vi "Open Waveform Sessions.vi"(8 "error in":errorcluster, 11 "Parameters":T4={"Name"="", "Rate.Hz"=0, "Injectors.Count"=0, "Injector.Timeout"=0.0, "Injector.Timer"=[], "Injector.Info"=[], "Events.Count"=[], "Event.Parameters"={"Shots"=0, "Shot.InitialVoltage"=0.0, "Shot.Stages"=0, "Stages"=[{"Stage.Dwell.Level"=0.0, "PullIn.Type"=enum."Pull In Transition Dwells", "PullIn.Level"=0.0, "Transition.Type"=enum."Stage Transition Voltage Level", "Transition.Level"=0.0}]}, "DMA.Ref"=refnum, "Waveform.Refs"=[], "Waveform.Sessions"=[], "Waveform.Enable"=refnum, "FPGA.Status"=refnum, "Search.Data"=refnum, "Results.Data"=refnum, "Results.Values"=[], "Results.Selections"=[]}) -> (0 "error out":errorcluster, 2 "Injection.Results":T1 {"Shots"."Results"."Off-Stage Avg Current" format="%#.6g"; "Shots"."Results"."Total Voltage Pulses" format="%#.6g"; "Shots"."Results"."Off-Stage Min Current" format="%#.6g"; "Shots"."Results"."Off-Stage Max Current" format="%#.6g"}, 3 "Parameters":T4={"Name"="", "Rate.Hz"=0, "Injectors.Count"=0, "Injector.Timeout"=0.0, "Injector.Timer"=[], "Injector.Info"=[], "Events.Count"=[], "Event.Parameters"={"Shots"=0, "Shot.InitialVoltage"=0.0, "Shot.Stages"=0, "Stages"=[{"Stage.Dwell.Level"=0.0, "PullIn.Type"=enum."Pull In Transition Dwells", "PullIn.Level"=0.0, "Transition.Type"=enum."Stage Transition Voltage Level", "Transition.Level"=0.0}]}, "DMA.Ref"=refnum, "Waveform.Refs"=[], "Waveform.Sessions"=[], "Waveform.Enable"=refnum, "FPGA.Status"=refnum, "Search.Data"=refnum, "Results.Data"=refnum, "Results.Values"=[], "Results.Selections"=[]})   [LabVIEW 2015, in "Fuel Injection Addon Engine.lvlib"]
uses:
  Fuel Injection Addon Engine.lvlib
  Types/Async Parameters.ctl
  Shared/Types/Injector info.ctl
  Shared/Types/Shot.Parameters.ctl
  Shared/Types/Stage.Parameters.ctl
  Shared/Types/Stage.PullIn.Types.ctl
  Shared/Types/Stage.Transition.Types.ctl
  <vilib>/NI Veristand/Custom Device API/Waveform Data Reference.ctl
  <vilib>/NI VeriStand/Custom Device Waveform API/Single Waveform Write (DBL)/Single Waveform Write (DBL).lvclass
  <vilib>/NI/NIVS Inline Async API/_Data Access Engine/Data Access Engine/Types/Read.DVR.ctl
  <vilib>/NI/NIVS Inline Async API/_Data Access Engine/Access Type Classes/Read/Read.lvclass
  <vilib>/NI/NIVS Inline Async API/_Data Access Engine/Data Access Engine/Types/Write.DVR.ctl
  <vilib>/NI/NIVS Inline Async API/_Data Access Engine/Access Type Classes/Write/Write.lvclass
  Shared/Types/Analysis.Channels.Select.ctl
  Types/Injector Event Data Cluster.ctl
  RT Analysis/Controls/Shot Information Control.ctl
  Types/Boost Stage Current Measurements Cluster Control.ctl
  <vilib>/NI Veristand/Custom Device Waveform API/Communication Properties.ctl
  <vilib>/NI Veristand/Custom Device Waveform API/Single Waveform Write (DBL)/NI VeriStand - Open Single Waveform Write Session (DBL).vi
  Shared/Constants.vi
  <vilib>/NI Veristand/Custom Device Waveform API/NI_VS Custom Device Waveform API.lvlib
  Shared/Fuel Injection Addon Shared.lvlib
  <vilib>/NI VeriStand/Custom Device API/Custom Device API.lvlib
  <vilib>/NI/NIVS Inline Async API/_Data Access Engine/Data Access Engine/Data Access Engine.lvclass
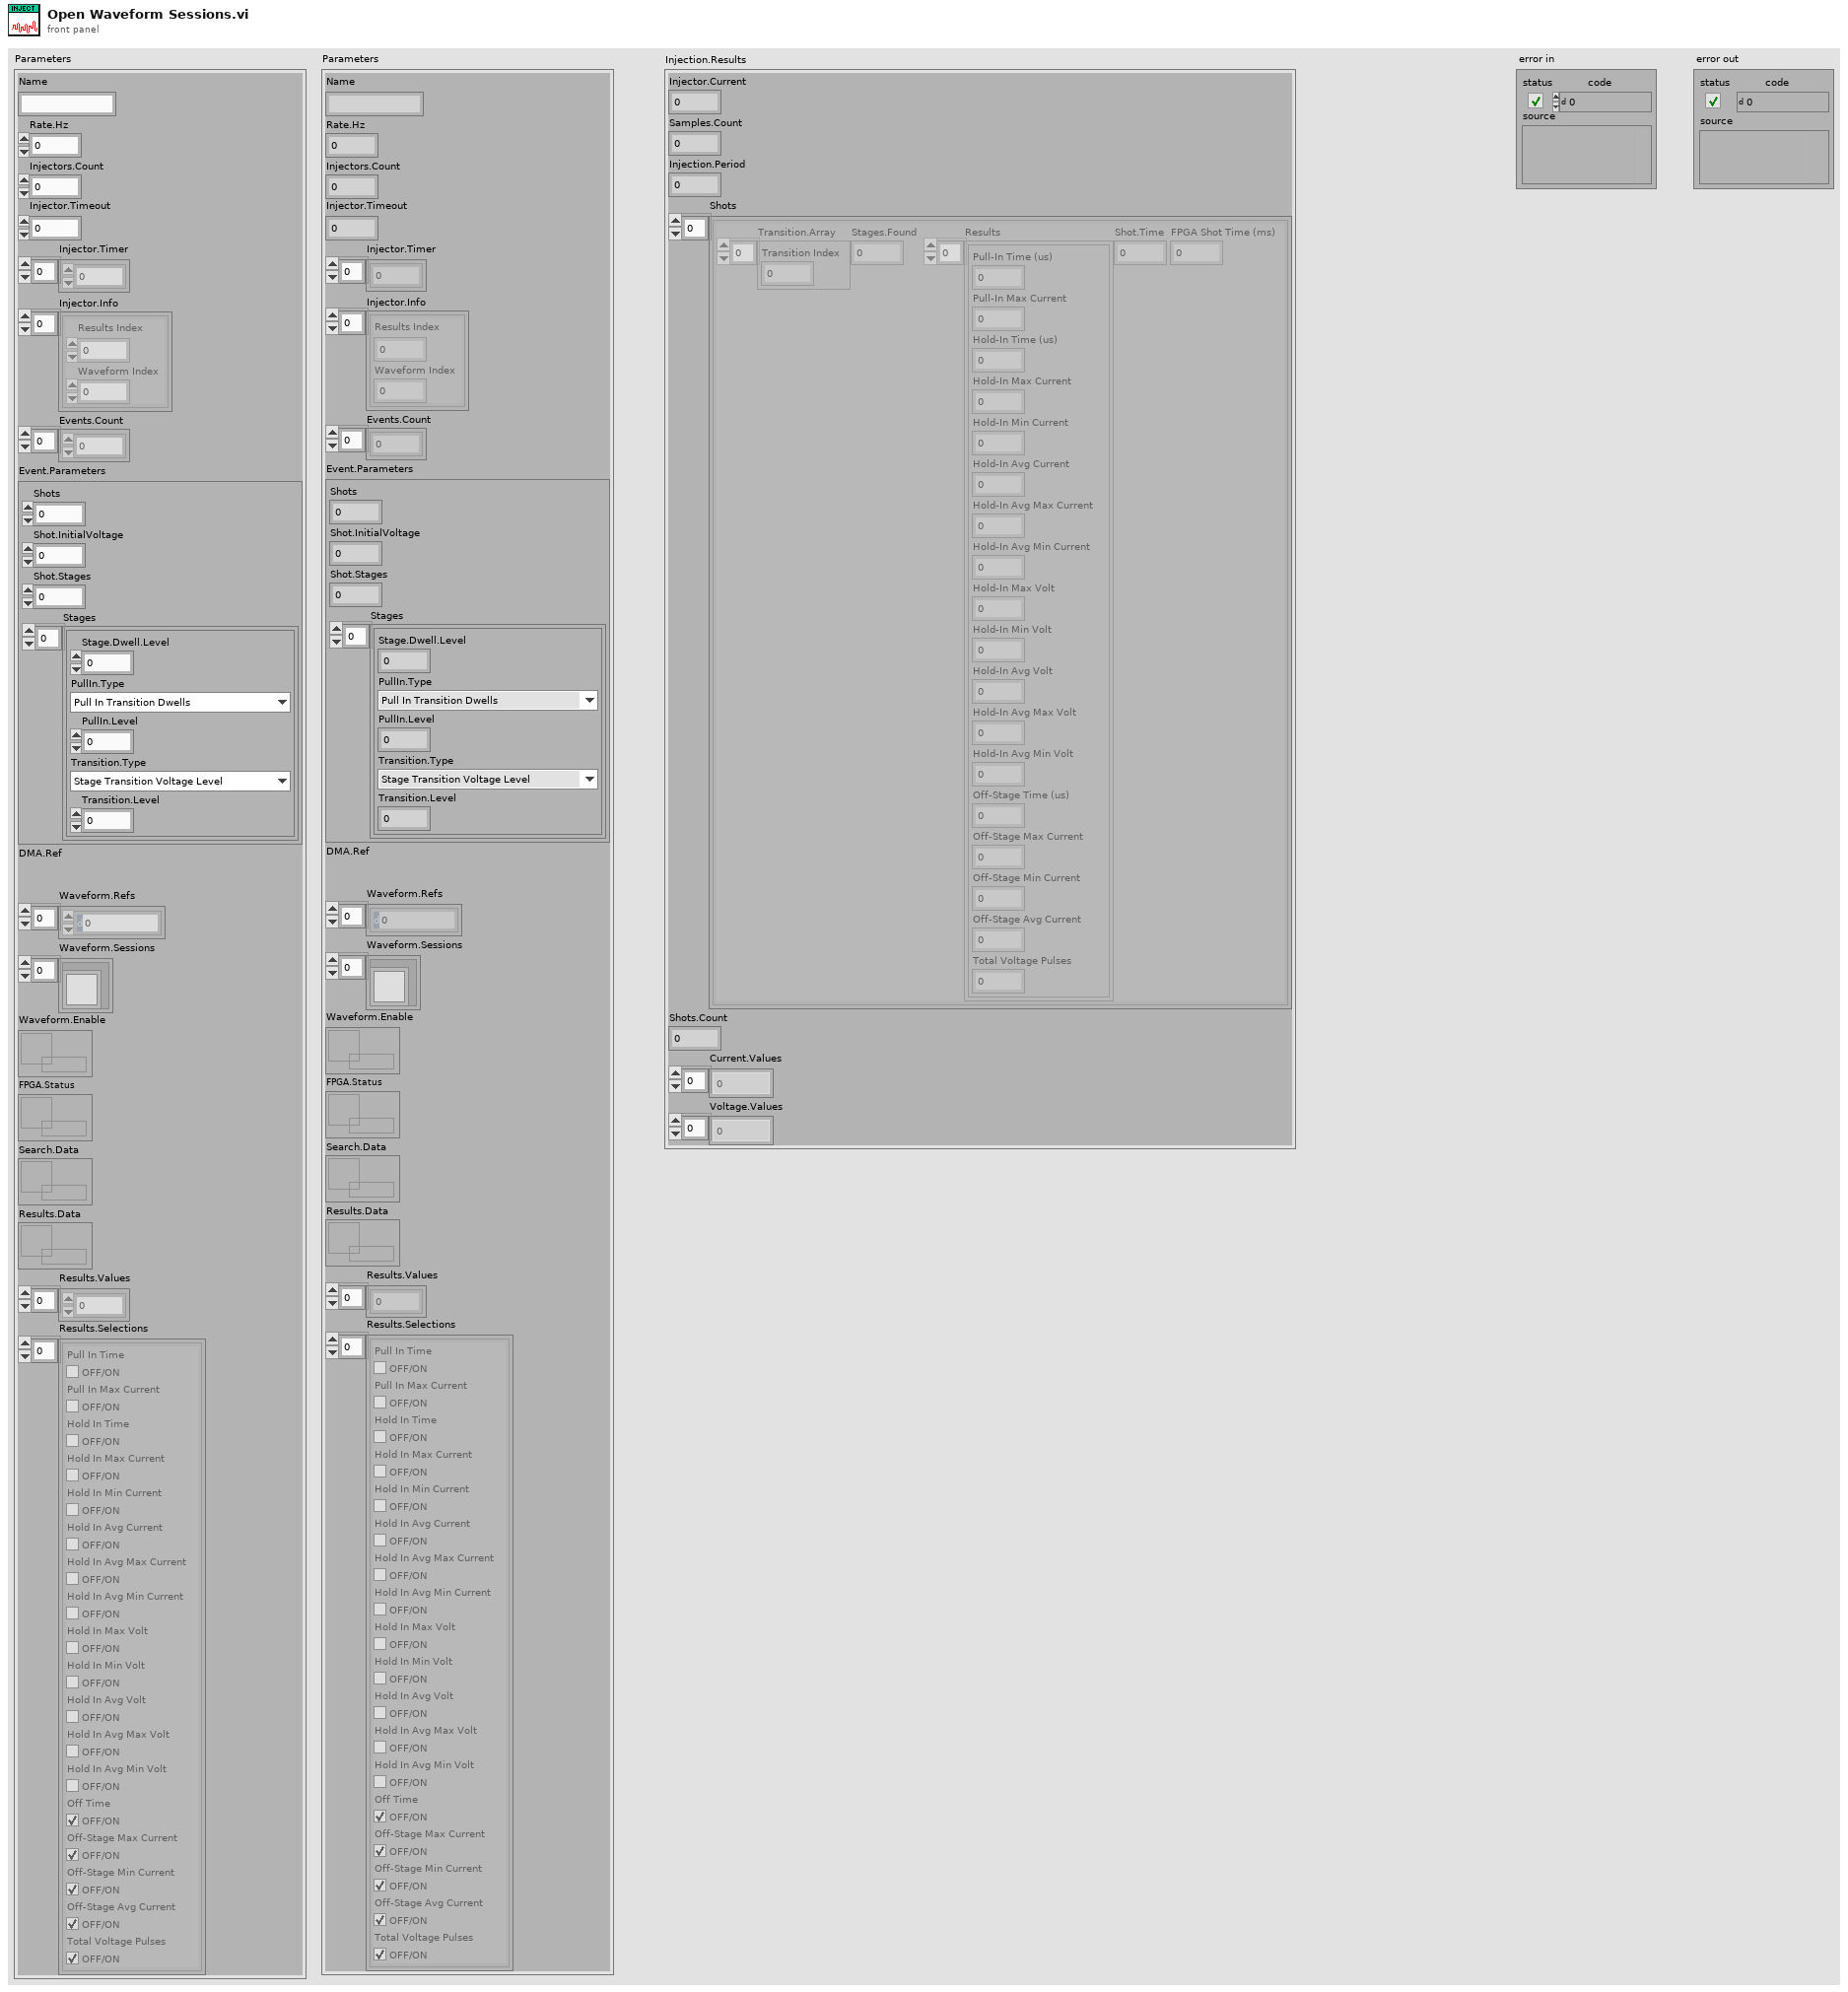
[diagram p1: front panel]
types:
  T1 = typedef "Fuel Injection Addon Engine.lvlib/Injector Event Data Cluster.ctl" = cluster{"Injector.Current":i16, "Samples.Count":i32, "Injection.Period":dbl, "Shots":T2[], "Shots.Count":i32, "Current.Values":dbl[], "Voltage.Values":dbl[]}
  T2 = typedef "Fuel Injection Addon Engine.lvlib/Shot Information Control.ctl" = cluster{"Transition.Array":i32[], "Stages.Found":u16, "Results":T3[], "Shot.Time":dbl, "FPGA Shot Time (ms)":dbl}
  T3 = typedef "Fuel Injection Addon Engine.lvlib/Boost Stage Current Measurements Cluster Control.ctl" = cluster{"Pull-In Time (us)":dbl, "Pull-In Max Current":dbl, "Hold-In Time (us)":dbl, "Hold-In Max Current":dbl, "Hold-In Min Current":dbl, "Hold-In Avg Current":dbl, "Hold-In Avg Max Current":dbl, "Hold-In Avg Min Current":dbl, "Hold-In Max Volt":dbl, "Hold-In Min Volt":dbl, "Hold-In Avg Volt":dbl, "Hold-In Avg Max Volt":dbl, "Hold-In Avg Min Volt":dbl, "Off-Stage Time (us)":dbl, "Off-Stage Max Current":dbl, "Off-Stage Min Current":dbl, "Off-Stage Avg Current":dbl, "Total Voltage Pulses":dbl}
  T4 = typedef "Fuel Injection Addon Engine.lvlib/Async Parameters.ctl" = cluster{"Name":string, "Rate.Hz":u32, "Injectors.Count":u8, "Injector.Timeout":dbl, "Injector.Timer":u32[], "Injector.Info":T5[], "Events.Count":u64[], "Event.Parameters":T6, "DMA.Ref":refnum<k20>, "Waveform.Refs":T10[], "Waveform.Sessions":refnum<class "Single Waveform Write (DBL).lvclass">[], "Waveform.Enable":T11, "FPGA.Status":T12, "Search.Data":T11, "Results.Data":T12, "Results.Values":dbl[], "Results.Selections":T13[]}
  T5 = typedef "Fuel Injection Addon Shared.lvlib/Injector info.ctl" = cluster{"Results Index":i32, "Waveform Index":i32}
  T6 = typedef "Fuel Injection Addon Shared.lvlib/Shot.Parameters.ctl" = cluster{"Shots":u32, "Shot.InitialVoltage":dbl, "Shot.Stages":u32, "Stages":T7[]}
  T7 = typedef "Fuel Injection Addon Shared.lvlib/Stage.Parameters.ctl" = cluster{"Stage.Dwell.Level":dbl, "PullIn.Type":T8, "PullIn.Level":dbl, "Transition.Type":T9, "Transition.Level":dbl}
  T8 = typedef "Stage.PullIn.Types.ctl" = enum8{"Pull In Transition Dwells", "Pull In Transition Current Drop"}
  T9 = typedef "Stage.Transition.Types.ctl" = enum8{"Stage Transition Dwell Time", "Stage Transition Voltage Level", "Stage Transition Current Drop"}
  T10 = typedef "Custom Device API.lvlib/Waveform Data Reference.ctl" = i32
  T11 = typedef "Data Access Engine.lvlib/Data Access Engine.lvclass/Read.DVR.ctl" = refnum<data-value>
  T12 = typedef "Data Access Engine.lvlib/Data Access Engine.lvclass/Write.DVR.ctl" = refnum<data-value>
  T13 = typedef "Fuel Injection Addon Shared.lvlib/Analysis.Channels.Select.ctl" = cluster{"Pull In Time":bool, "Pull In Max Current":bool, "Hold In Time":bool, "Hold In Max Current":bool, "Hold In Min Current":bool, "Hold In Avg Current":bool, "Hold In Avg Max Current":bool, "Hold In Avg Min Current":bool, "Hold In Max Volt":bool, "Hold In Min Volt":bool, "Hold In Avg Volt":bool, "Hold In Avg Max Volt":bool, "Hold In Avg Min Volt":bool, "Off Time":bool, "Off-Stage Max Current":bool, "Off-Stage Min Current":bool, "Off-Stage Avg Current":bool, "Total Voltage Pulses":bool}
  T14 = typedef "NI_VS Custom Device Waveform API.lvlib/Communication Properties.ctl" = cluster{"WPL":cluster{"Custom Queue Size":i32, "Use Custom Queue Size?":bool}}
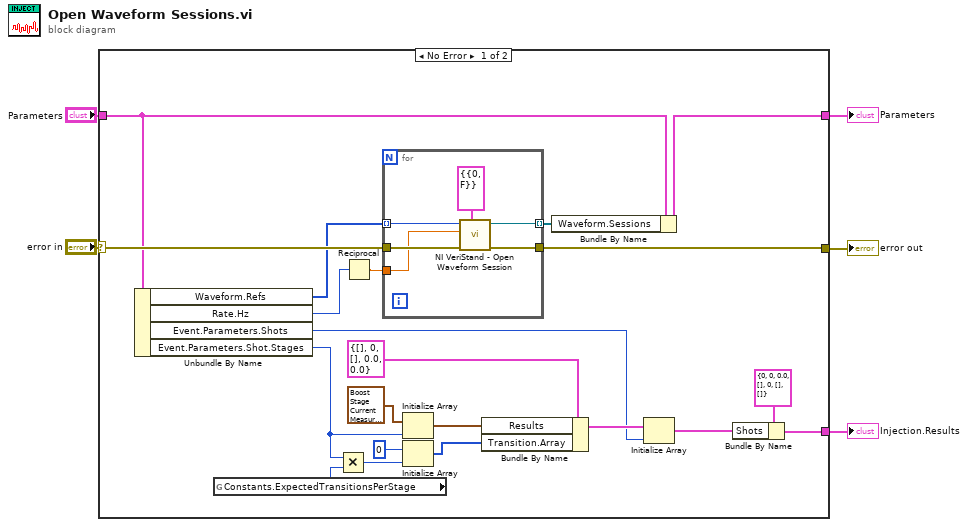
[diagram p0: block diagram]
diagram:
  n1 = case shown="No Error" "error in" {
    selector: "error in" -> [w26 w34]
    tunnel: "Parameters" -> [w23 w33]
    tunnel: [w25 w34] -> w4
    tunnel: [w22 w33] -> w2
    tunnel: [w11 _] -> w1
    frame No Error {
      n2 = Unbundle By Name(w23) -> ("Waveform.Refs"=w24:T10[], "Rate.Hz"=w20:u32, "Event.Parameters.Shots"=w13:u32, "Event.Parameters.Shot.Stages"=w10:u32)
      n3 = global read "Constants.vi" "Constants.ExpectedTransitionsPerStage"() -> (w6:u32)
      n4 = Multiply(x=w10, y=w6) -> (x*y=w9:u32)
      n5 = Reciprocal(x=w20) -> (1/x=w19:dbl)
      n6 = for {
        tunnel: w26 -> [w32]
        tunnel: [w31] -> w25
        tunnel: w24 -> [w30] mode=indexing
        tunnel: [w28] -> w21 mode=indexing
        tunnel: w19 -> [w27]
        n7 = call-poly <vilib>:"NI VeriStand - Open Waveform Session.vi"("Communication Properties"=T14 {"WPL"={"Custom Queue Size"=0, "Use Custom Queue Size?"=FALSE}}, "error in (no error)"=w32, "dt"=w27, "DBL Waveform Data Reference"=w30) -> ("error out"=w31:errorcluster, "Single Waveform Write Session (DBL)"=w28:refnum<class "Single Waveform Write (DBL).lvclass">)  [unwired: 6 in]
      }
      n8 = Initialize Array(T3 {"Pull-In Time (us)"=0.0, "Pull-In Max Current"=0.0, "Hold-In Time (us)"=0.0, "Hold-In Max Current"=0.0, "Hold-In Min Current"=0.0, "Hold-In Avg Current"=0.0, "Hold-In Avg Max Current"=0.0, "Hold-In Avg Min Current"=0.0, "Hold-In Max Volt"=0.0, "Hold-In Min Volt"=0.0, "Hold-In Avg Volt"=0.0, "Hold-In Avg Max Volt"=0.0, "Hold-In Avg Min Volt"=0.0, "Off-Stage Time (us)"=0.0, "Off-Stage Max Current"=0.0, "Off-Stage Min Current"=0.0, "Off-Stage Avg Current"=0.0, "Total Voltage Pulses"=0.0} ("Boost Stage Current Measurements"), w10) -> (w15:T3[])
      n9 = Initialize Array(0 ("Transition Index"), w9) -> (w7:i32[])
      n10 = Bundle By Name(cluster=T2 {"Transition.Array"=[], "Stages.Found"=0, "Results"=[], "Shot.Time"=0.0, "FPGA Shot Time (ms)"=0.0} ("Shot Info"), "Results"=w15, "Transition.Array"=w7) -> (w14:T2)
      n11 = Bundle By Name(cluster=w23, "Waveform.Sessions"=w21) -> (w22:T4)
      n12 = Initialize Array(w14, w13) -> (w12:T2[])
      n13 = Bundle By Name(cluster=T1 {"Injector.Current"=0, "Samples.Count"=0, "Injection.Period"=0.0, "Shots"=[], "Shots.Count"=0, "Current.Values"=[], "Voltage.Values"=[]} ("Injection Event Data Cluster in"), "Shots"=w12) -> (w11:T1)
    }
    frame Error {
    }
  }
  "error out" <- w4
  "Parameters" <- w2
  "Injection.Results" <- w1
